vi "Stop all measurements.vi"(8 "error in (no error)":errorcluster, 11 "Mag Lab Measure Controller in":refnum<class "Mag Lab Measure Controller.lvclass">) -> (0 "error out":errorcluster, 3 "Mag Lab Measure Controller out":refnum<class "Mag Lab Measure Controller.lvclass">)   [LabVIEW 2015, in "Mag Lab Measure Controller.lvclass"]
uses:
  Mag Lab Measure Controller.lvclass
  Mag Lab Measurement/Mag Lab Measurement.lvclass/Mag Lab Measurement.ctl
  Mag Lab Error Handler/Mag Lab Error Handler.lvclass
  Mag Lab Measurement/Mag Lab Measurement.lvclass
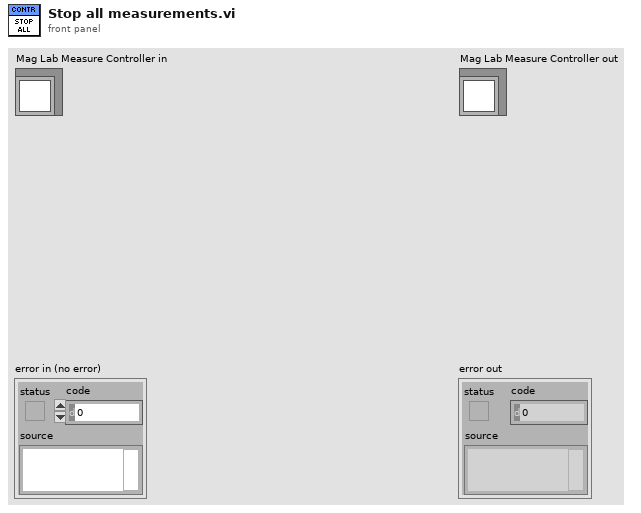
[diagram p1: front panel]
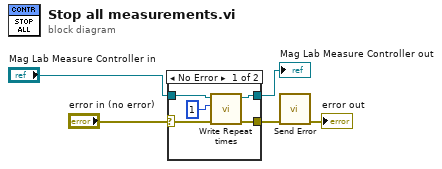
[diagram p0: block diagram]
diagram:
  n1 = case shown="No Error" "error in (no error)" {
    selector: "error in (no error)" -> [w7 w12]
    tunnel: [w10 w12] -> w4
    tunnel: [w9 w11] -> w2
    tunnel: "Mag Lab Measure Controller in" -> [w6 w11]
    frame No Error {
      n2 = call "Write Repeat times.vi"("error in (no error)"=w7, "Repeat times"=1, "Mag Lab Measurement in"=w6) -> ("error out"=w10:errorcluster, "Mag Lab Measurement out"=w9:refnum<class "Mag Lab Measure Controller.lvclass">)  [unwired: 7 in]
    }
    frame Error {
    }
  }
  "Mag Lab Measure Controller out" <- w2
  n3 = call "Send Error.vi"("error in (no error)"=w4) -> ("error out"=→"error out":errorcluster)  [unwired: 9 in, 1 out]
